vi "runJob.vi"(8 "error in (no error)":errorcluster, 10 "VGS_Job in":refnum<class "VGS_Job.lvclass">, 11 "VGS_RemoteControlClient in":refnum<class "VGS_RemoteControlClient.lvclass">) -> (0 "error out":errorcluster, 3 "VGS_RemoteControlClient out":refnum<class "VGS_RemoteControlClient.lvclass">)   [LabVIEW 2022 SP3, in "LV_VGS.lvlib" / "VGS_RemoteControlClient.lvclass"]
uses:
  VGS_RemoteControlClient.lvclass
  Job/VGS_Job.lvclass
  Job/VGS_Job.lvclass/VGS_Job.ctl
  VGS_RemoteControlClient.lvclass/VGS_RemoteControlClient.ctl
  C:/Users/Andrey/Desktop/hajo/LV_VGS/vgs_project.dll
  vgs_project.dll
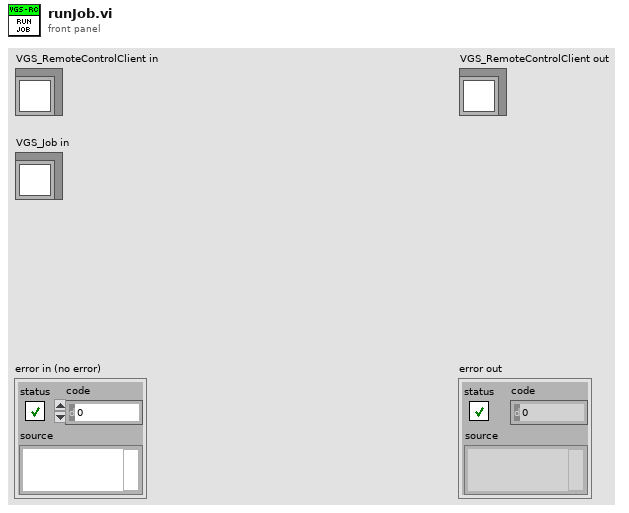
[diagram p1: front panel]
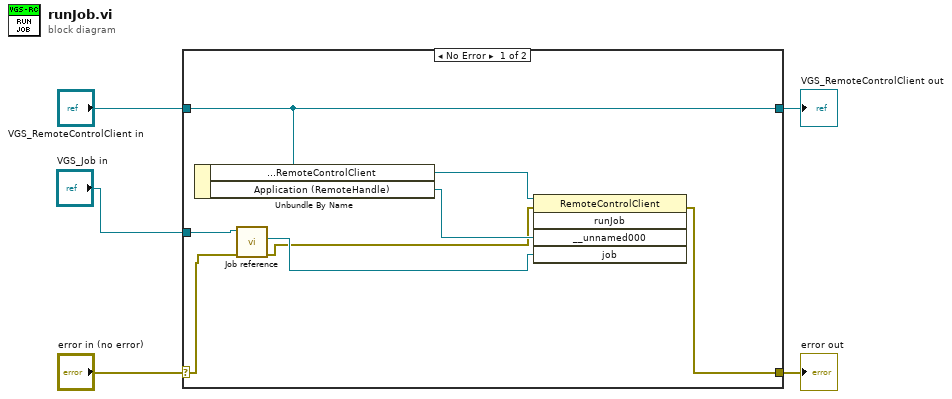
[diagram p0: block diagram]
diagram:
  n1 = case shown="No Error" "error in (no error)" {
    selector: "error in (no error)" -> [w7 w15]
    tunnel: [w11 w15] -> w4
    tunnel: [w13 w14] -> w2
    tunnel: "VGS_RemoteControlClient in" -> [w13 w14]
    tunnel: "VGS_Job in" -> [w9 _]
    frame No Error {
      n2 = Unbundle By Name(w13) -> ("VGS.Project.Interop.RemoteControlClient"=w12:refnum<k24>, "Application (RemoteHandle)"=w10:refnum<k24>)
      n3 = call "Job reference.vi"("error in (no error)"=w7, "VGS_Job in"=w9) -> ("error out"=w6:errorcluster, "Job reference"=w8:refnum<k24>)  [unwired: 7 in, 1 out]
      n4 = invoke class="RemoteControlClient" method="runJob"(reference=w12, error in=w6, "__unnamed000"=w10, "job"=w8) -> (error out=w11:errorcluster)  [unwired: 1 in, 4 out]
    }
    frame Error {
    }
  }
  "error out" <- w4
  "VGS_RemoteControlClient out" <- w2
